vi "Read Actor Ref.vi"(11 "Attributes in":refnum<class "Attributes.lvclass">) -> (2 "Actor Ref":refnum<vi>)   [LabVIEW 2025, in "jettl.lvlib" / "Attributes.lvlib" / "Attributes.lvclass"]
uses:
  Attributes.lvclass
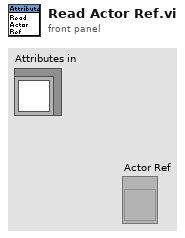
[diagram p1: front panel]
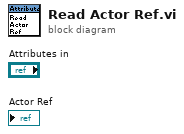
[diagram p0: block diagram]
diagram:
